vi "Pre Launch Init.vi"(11 "SLZ-KA1 in":refnum<class "SLZ-KA1.lvclass">) -> (0 "error out":errorcluster, 3 "SLZ-KA1 out":refnum<class "SLZ-KA1.lvclass">)   [LabVIEW 2015, in "SLZ-KA1 Actor.lvlib" / "SLZ-KA1.lvclass"]
doc: "(<B>Filename</B>: Actor Framework.lvlib:Actor.lvclass:Pre Launch Init.vi)\n\nDefines behavior that occurs after the Launch Nested Actor method is invoked but before the actor's Actor Core method begins running.\n\nBy default, this method does nothing. A descendant class may override it to define behavior."
uses:
  SLZ-KA1.lvclass
  Controls/SLZ-KA1 Real Data Cluster.ctl
  Controls/SLZ-KA1 Virtual Data Cluster.ctl
  SLZ-KA1.lvclass/SLZ-KA1.ctl
  <vilib>/ActorFramework/Actor/Actor.lvclass
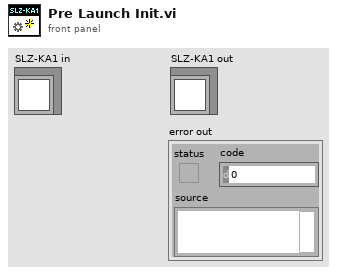
[diagram p1: front panel]
types:
  T1 = typedef "SLZ-KA1 Actor.lvlib/SLZ-KA1.lvclass/SLZ-KA1 Virtual Data Cluster.ctl" = cluster{"Drive Mode":u16, "Temperature Setpoint":dbl, "Drive On/Off":enum16{"Off", "On"}}
  T2 = typedef "SLZ-KA1 Actor.lvlib/SLZ-KA1.lvclass/SLZ-KA1 Real Data Cluster.ctl" = cluster{"Drive On/Off":enum16{"Off", "On"}, "Room Temperature":dbl, "Fault Code":u16}
  T3 = typedef "SLZ-KA1 Actor.lvlib/SLZ-KA1.lvclass/SLZ-KA1 Notifiers.ctl" = cluster{"stop":refnum<notifier>, "real data":refnum<notifier>, "virtual data":refnum<notifier>}
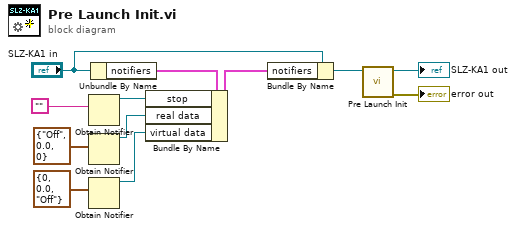
[diagram p0: block diagram]
diagram:
  n1 = Obtain Notifier(notification data type="") -> (notifier out=w8:refnum<notifier>)  [unwired: 3 in, 2 out]
  n2 = Obtain Notifier(notification data type=T2 {"Drive On/Off"=enum."Off", "Room Temperature"=0.0, "Fault Code"=0}) -> (notifier out=w4:refnum<notifier>)  [unwired: 3 in, 2 out]
  n3 = Obtain Notifier(notification data type=T1 {"Drive Mode"=0, "Temperature Setpoint"=0.0, "Drive On/Off"=enum."Off"} ("HVAC Data")) -> (notifier out=w1:refnum<notifier>)  [unwired: 3 in, 2 out]
  n4 = Unbundle By Name("SLZ-KA1 in") -> ("notifiers"=w7:T3)
  n5 = Bundle By Name(cluster=w7, "stop"=w8, "real data"=w4, "virtual data"=w1) -> (w6:T3)
  n6 = Bundle By Name(cluster="SLZ-KA1 in", "notifiers"=w6) -> (w11:refnum<class "SLZ-KA1.lvclass">)
  n7 = call-parent "Pre Launch Init.vi"("Actor in"=w11) -> ("error out"=→"error out":errorcluster, "Actor out"=→"SLZ-KA1 out":refnum<class "SLZ-KA1.lvclass">)  [unwired: 9 in]
